vi "PID Filter.vi"(3 "reinitialize? (F)":bool, 4 "input":dbl format="%.2f") -> (1 "output":dbl format="%.2f")   [LabVIEW 2011]
panel:
  # "same as the library version, except that, \nwhen it reinitializes, all values are set to 0, instead \nof retaining their previous values"
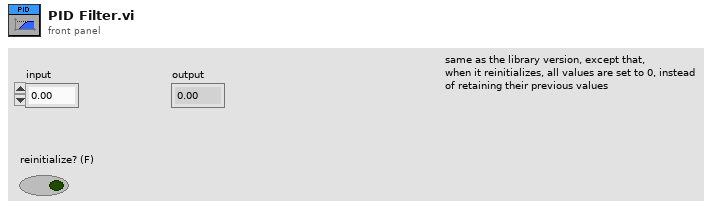
[diagram p1: front panel]
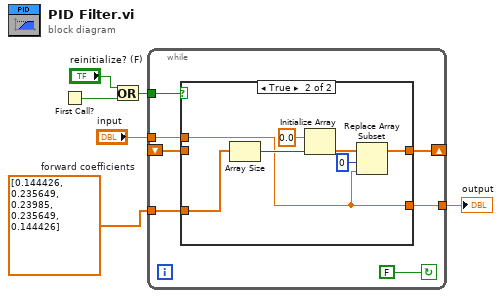
[diagram p0: block diagram]
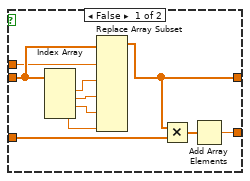
[diagram p2: hidden frame]
diagram:
  w3 = dbl[] [0.144426, 0.235649, 0.23985, 0.235649, 0.144426]  # forward coefficients
  n1 = First Call?() -> (First Call?: T/F=w1:bool)
  n2 = Or(x="reinitialize? (F)", y=w1) -> (x .or. y?=w6:bool)
  n3 = while {
    shift-left: _ -> [w9]
    shift-right: [w8] -> _
    tunnel: w6 -> [w10]
    tunnel: w3 -> [w11]
    tunnel: [w12] -> w4
    tunnel: "input" -> [w13]
    stop <- FALSE continue-if-true
    n4 = case shown="True" w10 {
      tunnel: w11 -> [w23 w29]
      tunnel: w9 -> [w20 _]
      tunnel: [w22 w24] -> w12
      tunnel: [w14 w26] -> w8
      tunnel: w13 -> [w19 w24]
      frame False {
        n5 = Index Array(array=w20) -> (element #1=w18:dbl, element #2=w17:dbl, element #3=w16:dbl, element #4=w15:dbl)  [unwired: 4 in]
        n6 = Replace Array Subset(array=w20, new element #1=w19, new element #2=w18, new element #3=w17, new element #4=w16, new element #5=w15) -> (w14:dbl[])  [unwired: 5 in]
        n7 = Multiply(x=w14, y=w23) -> (x*y=w21:dbl[])
        n8 = Add Array Elements(numeric array=w21) -> (sum=w22:dbl)
      }
      frame True {
        n9 = Array Size(array=w29) -> (size(s)=w30:i32)
        n10 = Initialize Array(0.0 ("element"), w30) -> (w27:dbl[])
        n11 = Replace Array Subset(array=w27, new element=w24, index=0) -> (w26:dbl[])
      }
    }
  }
  "output" <- w4
